vi "test_abs_conventional.vi"() -> ()   [LabVIEW 2017]
doc: "Minimal example that demonstrates functions implemented in the SorpPropLib for absorption working pairs based on the conventional approach."
panel:
  out "Der. of concentration wrt. pressure":cluster{dbl[], dbl[]}[](graph)
  out "Der. of concentration wrt. temperature":cluster{dbl[], dbl[]}[](graph)
  out "Der. of pressure wrt. concentration":cluster{dbl[], dbl[]}[](graph)
  out "Der. of pressure wrt. temperature":cluster{dbl[], dbl[]}[](graph)
  out "Temperature":cluster{dbl[], dbl[]}[](graph)
  out "Pressure":cluster{dbl[], dbl[]}[](graph)
  out "Concentration":cluster{dbl[], dbl[]}[](graph)
  in  "WorkingPair (Input)":T1={"no_iso"=1, "no_p_sat"=1, "path_db"="D:\\Driesel\\SorpLibLocal\\labview_wrapper\\data\\json\\sorpproplib.json", "wp_as"="NaOH-KOH-CsOH", "wp_st"="", "wp_iso"="Duehring", "wp_rf"="Water", "rf_rhol"="SaturatedLiquidDensity_EoS1", "no_rhol"=1, "rf_psat"="VaporPressure_EoS1"}
  in  "Temperature in K (Input)":dbl=300.0
  in  "Pressure in Pa (Input)":dbl=1000.0
  # "Increase pressure by 10 Pa in steps of 1 Pa."
  # "Path to database"
  # "Name of sorbent"
  # "Name of sub-type of sorbent"
  # "Name of refrigerant"
  # "Name of isotherm"
  # "ID of isotherm"
  # "Name of calculation approach for vapor pressure"
  # "ID of vapor pressure equation"
  # "Name of calculation approach for liquid density"
  # "ID of liquid density equation"
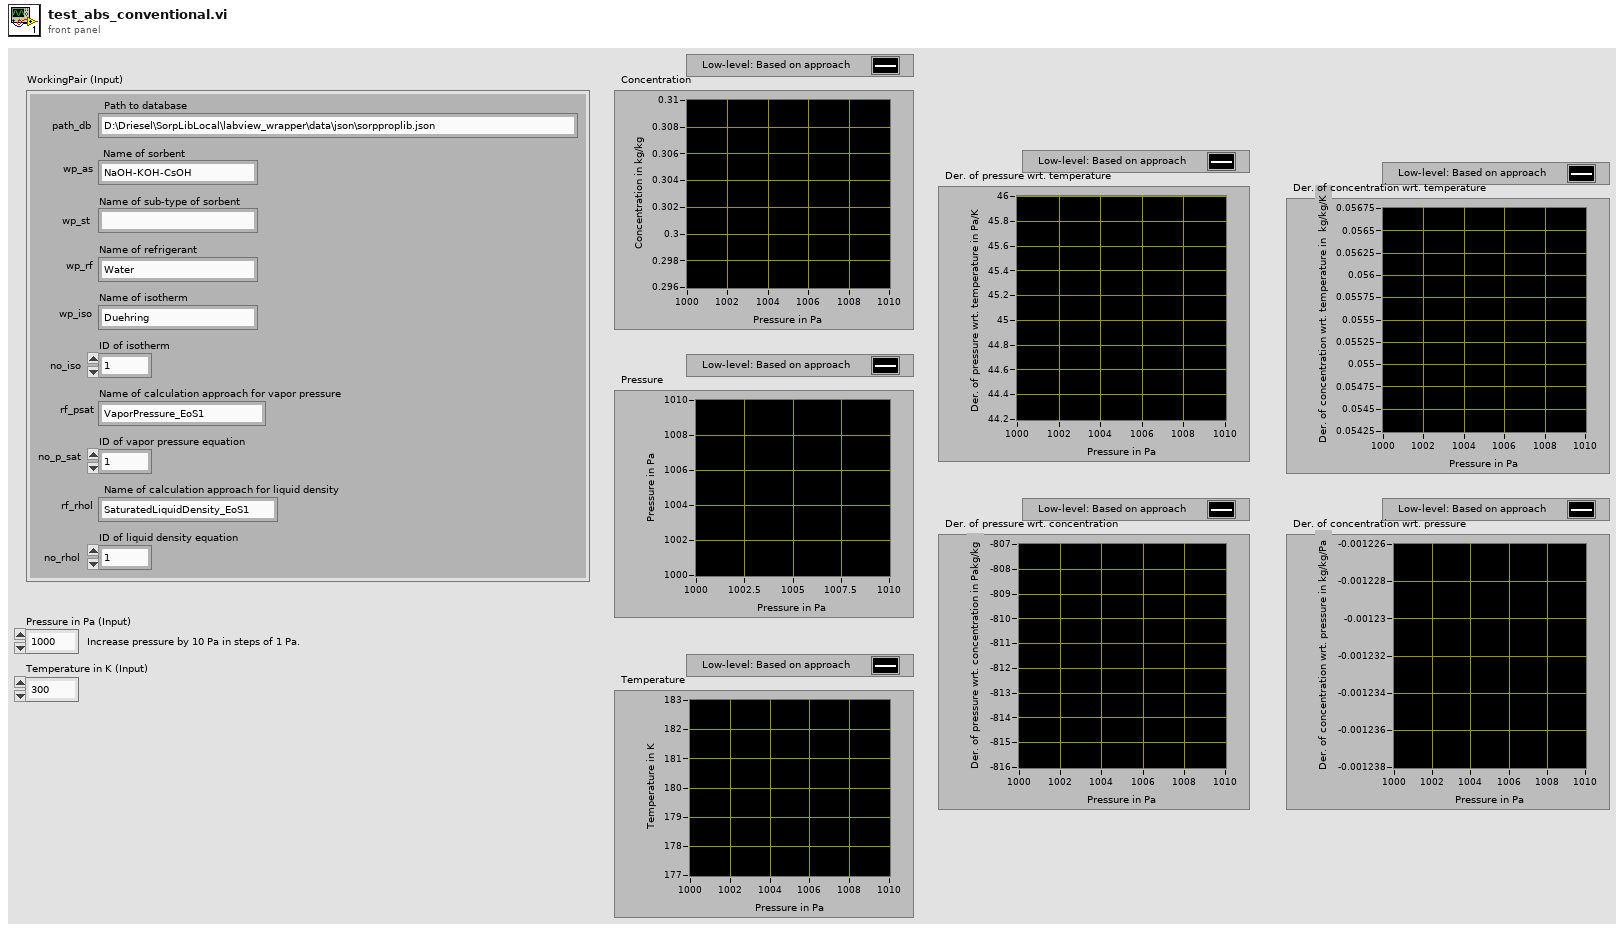
[diagram p1: front panel]
types:
  T1 = cluster{"no_iso":i32, "no_p_sat":i32, "path_db":string, "wp_as":string, "wp_st":string, "wp_iso":string, "wp_rf":string, "rf_rhol":string, "no_rhol":i32, "rf_psat":string}
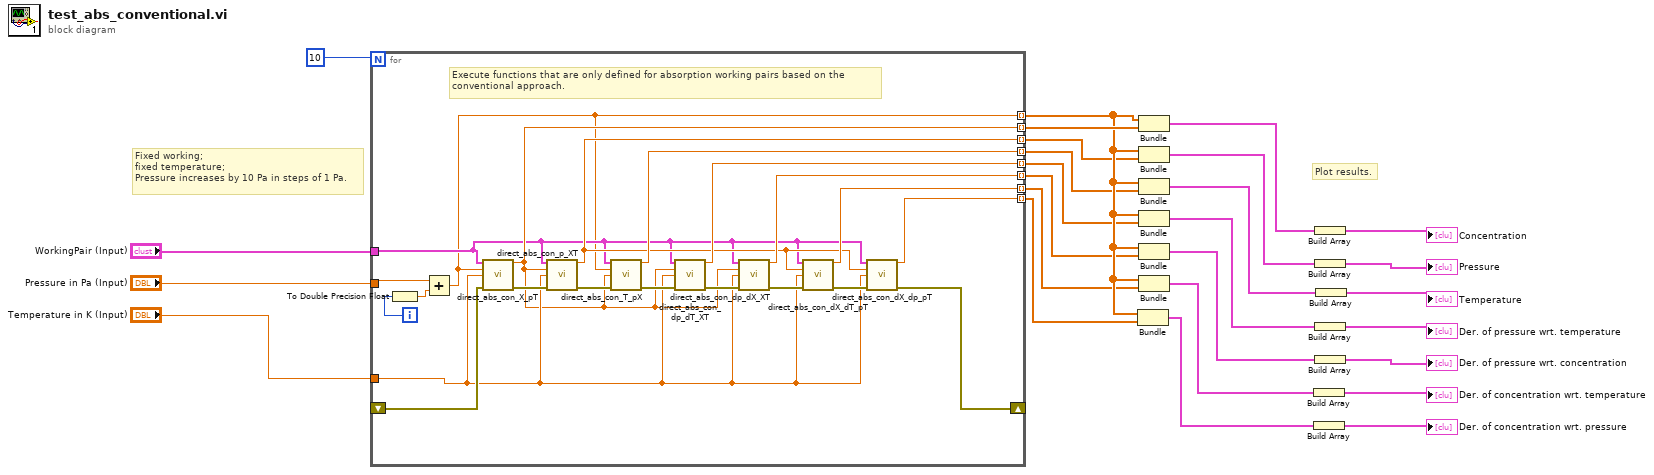
[diagram p0: block diagram]
diagram:
  # "Plot results."
  # "Fixed working;\nfixed temperature;\nPressure increases by 10 Pa in steps of 1 Pa."
  n1 = for {
    N: 10 -> [_]
    tunnel: "Pressure in Pa (Input)" -> [w47]
    tunnel: "Temperature in K (Input)" -> [w32]
    tunnel: "WorkingPair (Input)" -> [w28]
    shift-right: [w30] -> _
    shift-left: _ -> [w44]
    tunnel: [w42] -> w21 mode=indexing
    tunnel: [w27] -> w23 mode=indexing
    tunnel: [w29] -> w24 mode=indexing
    tunnel: [w33] -> w22 mode=indexing
    tunnel: [w40] -> w20 mode=indexing
    tunnel: [w38] -> w19 mode=indexing
    tunnel: [w35] -> w17 mode=indexing
    tunnel: [w31] -> w18 mode=indexing
    i -> [w46]
    # "Execute functions that are only defined for absorption working pairs based on the\nconventional approach."
    n2 = To Double Precision Float(number=w46) -> (double precision float=w45:dbl)
    n3 = Add(x=w47, y=w45) -> (x+y=w27:dbl)
    n4 = call "direct_abs_con_X_pT.vi"("WorkingPair (Input)"=w28, "Pressure in Pa (Input)"=w27, "Temperature in K (Input)"=w32, "Error (Input)"=w44) -> ("Concentration in kg/kg (Output)"=w29:dbl, "Error (Output)"=w43:errorcluster)  [unwired: 10 in]
    n5 = call "direct_abs_con_p_XT.vi"("WorkingPair (Input)"=w28, "Concentration in kg/kg (Input)"=w29, "Temperature in K (Input)"=w32, "Error (Input)"=w43) -> ("Pressure in Pa (Output)"=w33:dbl, "Error (Output)"=w41:errorcluster)  [unwired: 10 in]
    n6 = call "direct_abs_con_T_pX.vi"("WorkingPair (Input)"=w28, "Pressure in Pa (Input)"=w27, "Concentration in kg/kg (Input)"=w29, "Error (Input)"=w41) -> ("Temperature in K (Output)"=w42:dbl, "Error (Output)"=w39:errorcluster)  [unwired: 10 in]
    n7 = call "direct_abs_con_dp_dT_XT.vi"("WorkingPair (Input)"=w28, "Concentration in kg/kg (Input)"=w29, "Temperature in K (Input)"=w32, "Error (Input)"=w39) -> ("Der. of equilibrium pressure wrt. temperature in Pa/K (Output)"=w40:dbl, "Error (Output)"=w37:errorcluster)  [unwired: 10 in]
    n8 = call "direct_abs_con_dp_dX_XT.vi"("WorkingPair (Input)"=w28, "Concentration in kg/kg (Input)"=w29, "Temperature in K (Input)"=w32, "Error (Input)"=w37) -> ("Der. of equilibrium pressure wrt. concentration in Pakg/kg (Output)"=w38:dbl, "Error (Output)"=w36:errorcluster)  [unwired: 10 in]
    n9 = call "direct_abs_con_dX_dT_pT.vi"("WorkingPair (Input)"=w28, "Pressure in Pa (Input)"=w33, "Temperature in K (Input)"=w32, "Error (Input)"=w36) -> ("Der. of equilibrium concentration wrt. temperature in kg/kg/K (Output)"=w35:dbl, "Error (Output)"=w34:errorcluster)  [unwired: 10 in]
    n10 = call "direct_abs_con_dX_dp_pT.vi"("WorkingPair (Input)"=w28, "Pressure in Pa (Input)"=w33, "Temperature in K (Input)"=w32, "Error (Input)"=w34) -> ("Der. of equilibrium concentration wrt. pressure in kg/kg/Pa (Output)"=w31:dbl, "Error (Output)"=w30:errorcluster)  [unwired: 10 in]
  }
  n11 = Bundle(w23, w18) -> (w5:cluster{dbl[], dbl[]})  [unwired: 1 in]
  n12 = Bundle(w23, w24) -> (w16:cluster{dbl[], dbl[]})  [unwired: 1 in]
  n13 = Bundle(w23, w22) -> (w15:cluster{dbl[], dbl[]})  [unwired: 1 in]
  n14 = Bundle(w23, w21) -> (w14:cluster{dbl[], dbl[]})  [unwired: 1 in]
  n15 = Bundle(w23, w20) -> (w13:cluster{dbl[], dbl[]})  [unwired: 1 in]
  n16 = Bundle(w23, w19) -> (w8:cluster{dbl[], dbl[]})  [unwired: 1 in]
  n17 = Bundle(w23, w17) -> (w6:cluster{dbl[], dbl[]})  [unwired: 1 in]
  n18 = Build Array(w6) -> (→"Der. of concentration wrt. temperature":cluster{dbl[], dbl[]}[])
  n19 = Build Array(w5) -> (→"Der. of concentration wrt. pressure":cluster{dbl[], dbl[]}[])
  n20 = Build Array(w16) -> (→"Concentration":cluster{dbl[], dbl[]}[])
  n21 = Build Array(w15) -> (→"Pressure":cluster{dbl[], dbl[]}[])
  n22 = Build Array(w13) -> (→"Der. of pressure wrt. temperature":cluster{dbl[], dbl[]}[])
  n23 = Build Array(w8) -> (→"Der. of pressure wrt. concentration":cluster{dbl[], dbl[]}[])
  n24 = Build Array(w14) -> (→"Temperature":cluster{dbl[], dbl[]}[])
